vi "JJMCclase5.vi"() -> ()   [LabVIEW 2011]
panel:
  in  "Seleccionador Local":i32(ring) items=["Local 1", "Local 2", "Local 3"]
  out "A/C":bool
  out "Numero Personas":i32
  out "temperatura":i32(slide) scale=0.0..100.0
  # "Debemos seleccionar el local luego generar el numero de personas entre 1-60. El A/C se enciende de \nacuerdo a los lisguientes casos:\nLocal   Condicion para encender el A/C\nLocal 1  Si la temperatura es mayor a 25 o el numero de empleados es mayor a 30\nLocal 2  Si la temperatura es mayor a 28 o el numero de empleados es mayor a 35\nLocal 3  Si la temperatura es mayor a 24 o el numero de empleados es mayor a 20"
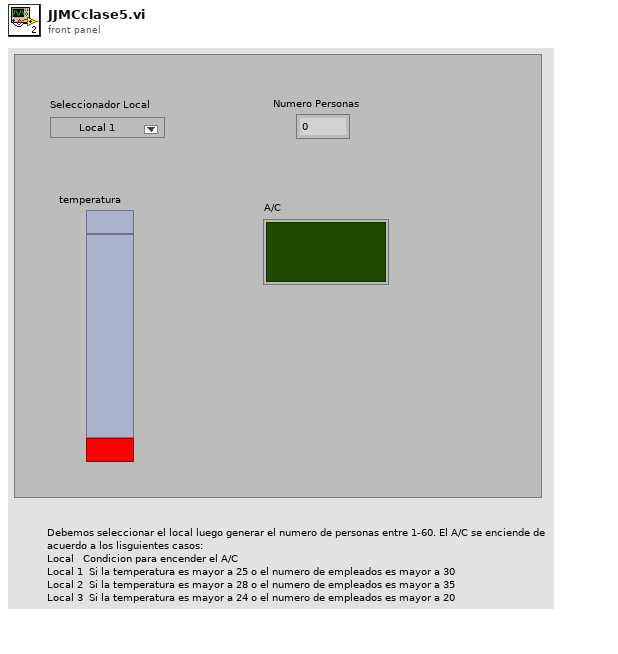
[diagram p1: front panel]
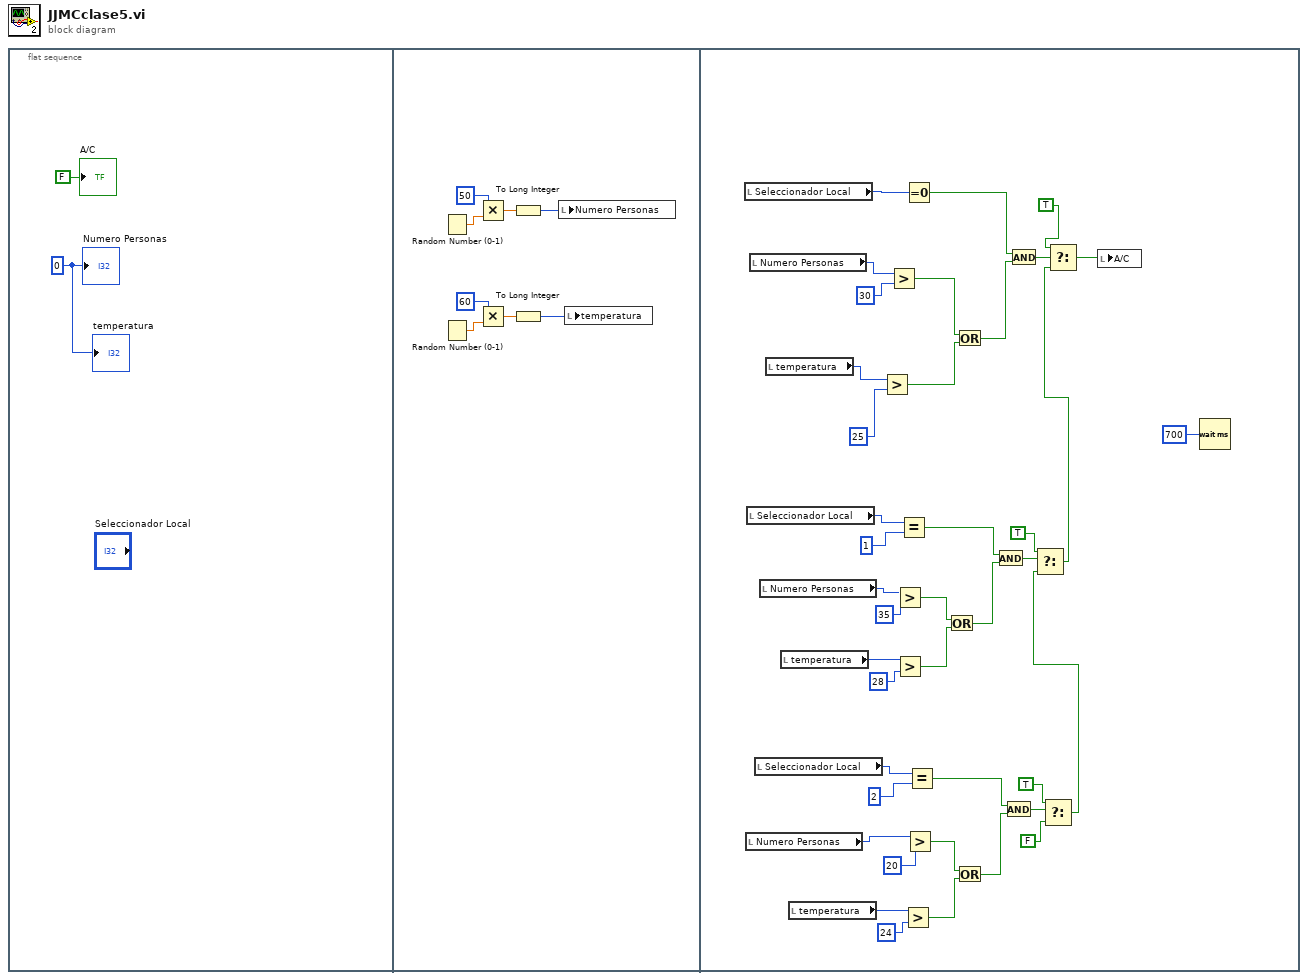
[diagram p0: block diagram]
diagram:
  n1 = flat-sequence {
    frame #0 {
      w1 = 0
      "temperatura" <- w1
      "Numero Personas" <- w1
      "A/C" <- FALSE ("A/C")
    }
    frame #1 {
      n2 = Random Number (0-1)() -> (number: 0 to 1=w9:dbl)
      n3 = Random Number (0-1)() -> (number: 0 to 1=w6:dbl)
      n4 = Multiply(x=50, y=w9) -> (x*y=w10:dbl)
      n5 = Multiply(x=60, y=w6) -> (x*y=w5:dbl)
      n6 = To Long Integer(number=w10) -> (32bit integer=w3:i32)
      n7 = To Long Integer(number=w5) -> (32bit integer=w4:i32)
      n8 = local write "Numero Personas"(w3) -> ()
      n9 = local write "temperatura"(w4) -> ()
    }
    frame #2 {
      n10 = local read "Seleccionador Local"() -> (w50:i32)
      n11 = local read "Numero Personas"() -> (w15:i32)
      n12 = local read "Seleccionador Local"() -> (w37:i32)
      n13 = local read "Numero Personas"() -> (w48:i32)
      n14 = local read "Seleccionador Local"() -> (w21:i32)
      n15 = local read "Numero Personas"() -> (w17:i32)
      n16 = local read "temperatura"() -> (w47:i32)
      n17 = local read "temperatura"() -> (w36:i32)
      n18 = local read "temperatura"() -> (w22:i32)
      n19 = Greater?(x=w47, y=25) -> (0:w44:bool)
      n20 = Greater?(x=w48, y=30) -> (0:w45:bool)
      n21 = Greater?(x=w17, y=35) -> (0:w16:bool)
      n22 = Greater?(x=w36, y=28) -> (0:w34:bool)
      n23 = Equal?(x=w37, y=1) -> (x = y?=w33:bool)
      n24 = Greater?(x=w22, y=24) -> (0:w24:bool)
      n25 = Equal To 0?(x=w50) -> (x = 0?=w42:bool)
      n26 = Greater?(x=w15, y=20) -> (0:w13:bool)
      n27 = Equal?(x=w21, y=2) -> (x = y?=w25:bool)
      n28 = Or(x=w16, y=w34) -> (x .or. y?=w32:bool)
      n29 = Or(x=w45, y=w44) -> (x .or. y?=w43:bool)
      n30 = Or(x=w13, y=w24) -> (x .or. y?=w26:bool)
      n31 = And(x=w33, y=w32) -> (x .and. y?=w31:bool)
      n32 = And(x=w25, y=w26) -> (x .and. y?=w27:bool)
      n33 = And(x=w42, y=w43) -> (x .and. y?=w41:bool)
      n34 = Select(t=TRUE, s=w27, f=FALSE) -> (s? t:f=w19:bool)
      n35 = Select(t=TRUE, s=w31, f=w19) -> (s? t:f=w30:bool)
      n36 = Select(t=TRUE, s=w41, f=w30) -> (s? t:f=w39:bool)
      n37 = local write "A/C"(w39) -> ()
      n38 = Wait (ms)(milliseconds to wait=700) -> ()  [unwired: 1 out]
    }
  }
